vi "Symphony Setup V2.vi"(4 "areas :":i32[][](array[numeric])=[[1], [1], [1], [1024], [256], [1], [1]], 5 "Function":T1, 6 "Acq type":i32(ring)=1 items=["JYMCD_ACQ_FORMAT_IMAGE", "JYMCD_ACQ_FORMAT_SCAN"], 7 "Int_time(ms)":u16=10 caption="Integration time(ms)", 8 "error in (no error)":errorcluster, 9 "Gain":i32, 10 "Select ADC":i32(ring) items=["JY_ADC_16_BIT", "JY_ADC_14_BIT", "JY_ADC_18_BIT"], 11 "JYCCDLib.IJYCCDReqd":refnum<k7>) -> (0 "error out":errorcluster, 1 "DataSize":i32, 3 "JYCCDLib.IJYCCDReqdOut":refnum<k7>)   [LabVIEW 2019]
uses:
  AcqParState.ctl
panel:
  # "Area#"
  # "X Origin"
  # "Y Origin"
  # "X Size"
  # "Y Size"
  # "X Bin"
  # "Y Bin"
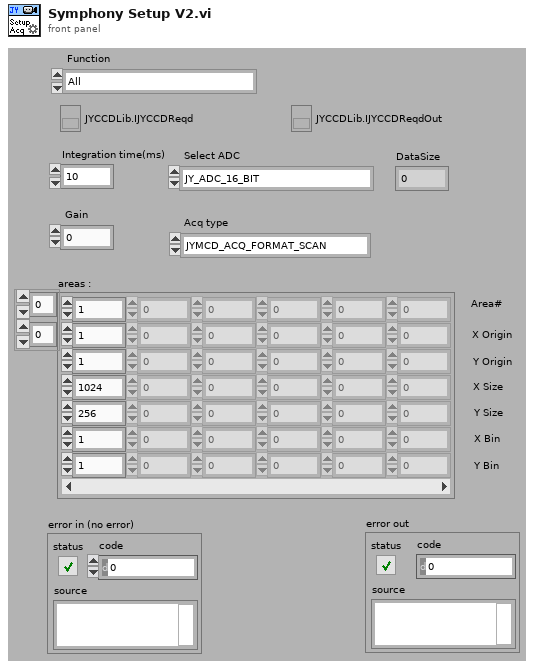
[diagram p1: front panel]
types:
  T1 = typedef "AcqParState.ctl" = enum16{"All", "ADC", "Gain", "AcqType", "IntegTime", "Areas", "Error"}
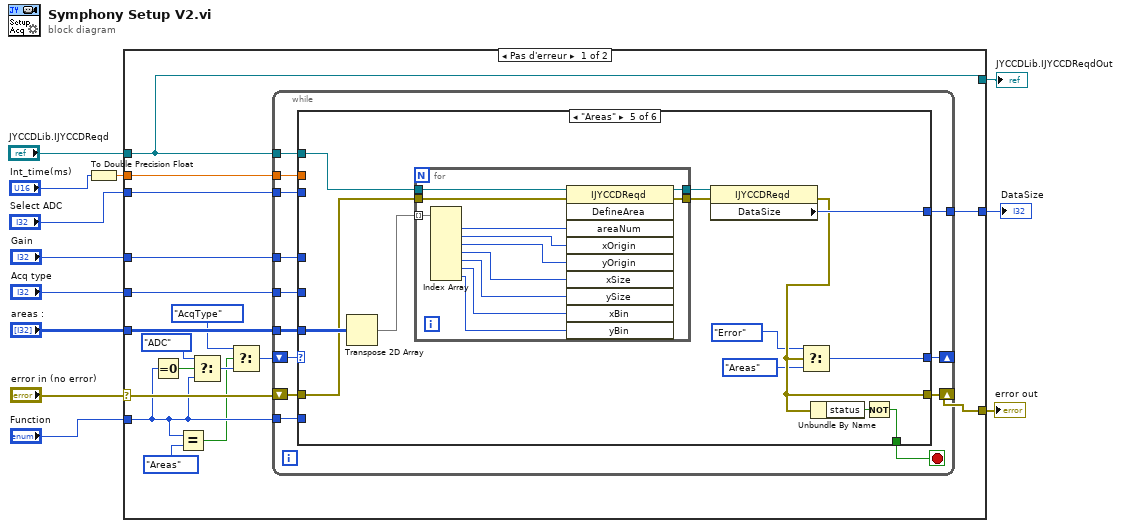
[diagram p0: block diagram]
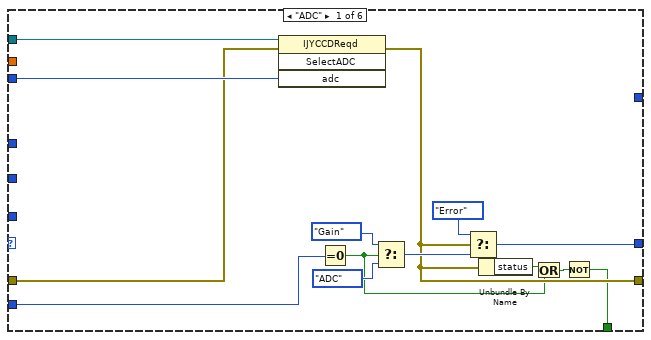
[diagram p2: hidden frame]
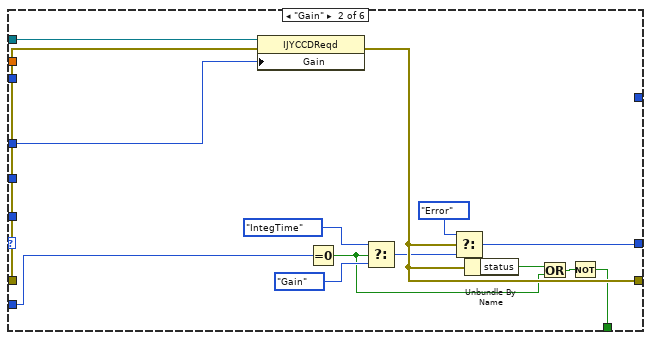
[diagram p3: hidden frame]
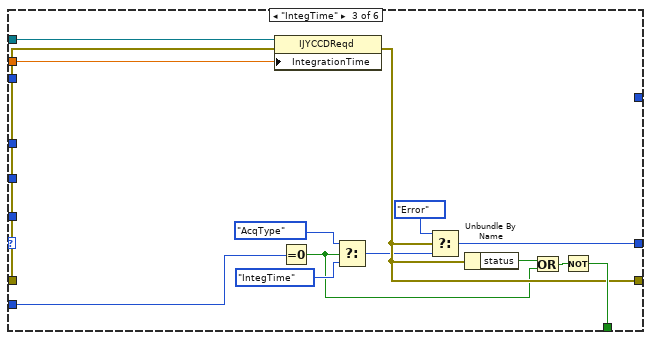
[diagram p4: hidden frame]
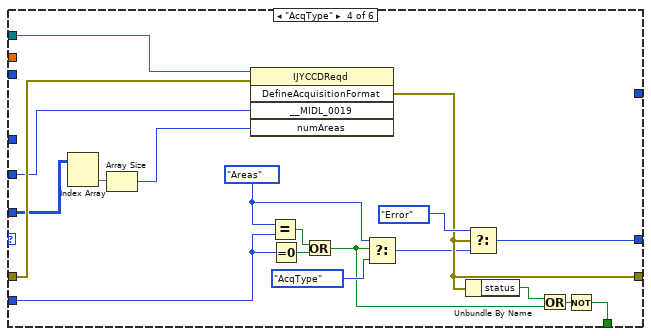
[diagram p5: hidden frame]
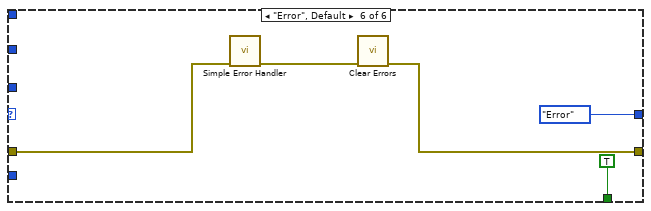
[diagram p6: hidden frame]
diagram:
  n1 = To Double Precision Float(number="Int_time(ms)") -> (double precision float=w8:dbl)
  n2 = case shown="Pas d'erreur" "error in (no error)" {
    selector: "error in (no error)" -> [w29 w135]
    tunnel: [w28 w135] -> w11
    tunnel: "JYCCDLib.IJYCCDReqd" -> [w25 w134]
    tunnel: w8 -> [w27 _]
    tunnel: "Select ADC" -> [w26 _]
    tunnel: [w25 w134] -> w6
    tunnel: "Gain" -> [w24 _]
    tunnel: "Acq type" -> [w23 _]
    tunnel: "areas :" -> [w22 _]
    tunnel: [w21 _] -> w2
    tunnel: "Function" -> [w17 _]
    frame No Error {
      n3 = Equal To 0?(x=w17) -> (x = 0?=w20:bool)
      n4 = Equal?(x=w17, y=AcqParState."Areas" ("Function")) -> (x = y?=w14:bool)
      n5 = Select(t=AcqParState."ADC" ("Function"), s=w20, f=w17) -> (s? t:f=w16:T1)
      n6 = Select(t=AcqParState."AcqType" ("Function"), s=w14, f=w16) -> (s? t:f=w15:T1)
      n7 = while {
        shift-right: [w38] -> w28
        shift-left: w29 -> [w41]
        tunnel: w25 -> [w42]
        shift-right: [w34] -> _
        shift-left: w15 -> [w30]
        tunnel: w27 -> [w40]
        tunnel: w26 -> [w39]
        tunnel: w24 -> [w37]
        tunnel: w23 -> [w36]
        tunnel: w22 -> [w35]
        tunnel: [w32] -> w21
        tunnel: w17 -> [w31]
        stop <- w33 stop-if-true
        n8 = case shown="\"Areas\"" w30 {
          tunnel: w42 -> [w53 w68 w83 w100 w105 _]
          tunnel: w41 -> [w54 w69 w84 w101 w104 w133]
          tunnel: w40 -> [_ _ w82 _ _ _]
          tunnel: w39 -> [w56 _ _ _ _ _]
          tunnel: [w47 w61 w76 w94 w109 w130] -> w38
          tunnel: w37 -> [_ w70 _ _ _ _]
          tunnel: w36 -> [_ _ _ w97 _ _]
          tunnel: w35 -> [_ _ _ w98 w108 _]
          tunnel: [w55 w58 w77 w103 w113 AcqParState."Error" ("Function")] -> w34
          tunnel: [w43 w57 w78 w102 w111 TRUE] -> w33
          tunnel: [_ _ _ _ w110 _] -> w32
          tunnel: w31 -> [w52 w66 w71 w90 _ _]
          frame "ADC" {
            n9 = invoke class="IJYCCDReqd" method="SelectADC"(reference=w53, error in=w54, "adc"=w56) -> (error out=w47:errorcluster)  [unwired: 1 in, 3 out]
            n10 = Equal To 0?(x=w52) -> (x = 0?=w45:bool)
            n11 = Select(t=AcqParState."Gain" ("Function"), s=w45, f=AcqParState."ADC" ("Function")) -> (s? t:f=w49:T1)
            n12 = Select(t=AcqParState."Error" ("Function"), s=w47, f=w49) -> (s? t:f=w55:T1)
            n13 = Unbundle By Name(w47) -> ("status"=w46:bool)
            n14 = Or(x=w46, y=w45) -> (x .or. y?=w44:bool)
            n15 = Not(x=w44) -> (.not. x?=w43:bool)
          }
          frame "Gain" {
            n16 = property class="IJYCCDReqd"(reference=w68, error in=w69, "Gain"=w70) -> (error out=w61:errorcluster)  [unwired: 1 out]
            n17 = Equal To 0?(x=w66) -> (x = 0?=w60:bool)
            n18 = Select(t=AcqParState."IntegTime" ("Function"), s=w60, f=AcqParState."Gain" ("Function")) -> (s? t:f=w59:T1)
            n19 = Select(t=AcqParState."Error" ("Function"), s=w61, f=w59) -> (s? t:f=w58:T1)
            n20 = Unbundle By Name(w61) -> ("status"=w63:bool)
            n21 = Or(x=w63, y=w60) -> (x .or. y?=w62:bool)
            n22 = Not(x=w62) -> (.not. x?=w57:bool)
          }
          frame "IntegTime" {
            n23 = property class="IJYCCDReqd"(reference=w83, error in=w84, "IntegrationTime"=w82) -> (error out=w76:errorcluster)  [unwired: 1 out]
            n24 = Equal To 0?(x=w71) -> (x = 0?=w73:bool)
            n25 = Select(t=AcqParState."AcqType" ("Function"), s=w73, f=AcqParState."IntegTime" ("Function")) -> (s? t:f=w72:T1)
            n26 = Select(t=AcqParState."Error" ("Function"), s=w76, f=w72) -> (s? t:f=w77:T1)
            n27 = Unbundle By Name(w76) -> ("status"=w80:bool)
            n28 = Or(x=w80, y=w73) -> (x .or. y?=w79:bool)
            n29 = Not(x=w79) -> (.not. x?=w78:bool)
          }
          frame "AcqType" {
            w91 = AcqParState."Areas" ("Function")
            n30 = Index Array(array=w98) -> (element=w99:i32[])  [unwired: 2 in]
            n31 = Array Size(array=w99) -> (size(s)=w96:i32)
            n32 = invoke class="IJYCCDReqd" method="DefineAcquisitionFormat"(reference=w100, error in=w101, "__MIDL_0019"=w97, "numAreas"=w96) -> (error out=w94:errorcluster)  [unwired: 1 in, 4 out]
            n33 = Equal?(x=w91, y=w90) -> (x = y?=w92:bool)
            n34 = Equal To 0?(x=w90) -> (x = 0?=w93:bool)
            n35 = Or(x=w92, y=w93) -> (x .or. y?=w87:bool)
            n36 = Select(t=w91, s=w87, f=AcqParState."AcqType" ("Function")) -> (s? t:f=w86:T1)
            n37 = Unbundle By Name(w94) -> ("status"=w85:bool)
            n38 = Select(t=AcqParState."Error" ("Function"), s=w94, f=w86) -> (s? t:f=w103:T1)
            n39 = Or(x=w85, y=w87) -> (x .or. y?=w88:bool)
            n40 = Not(x=w88) -> (.not. x?=w102:bool)
          }
          frame "Areas" {
            n41 = Transpose 2D Array(2D array=w108) -> (transposed array=w116:i32[][])
            n42 = for {
              tunnel: [w127] -> w114
              tunnel: [w126] -> w115
              tunnel: w116 -> [w125] mode=indexing
              tunnel: w104 -> [w118]
              tunnel: w105 -> [w117]
              n43 = Index Array(array=w125) -> (element #1=w128:i32, element #2=w124:i32, element #3=w123:i32, element #4=w122:i32, element #5=w121:i32, element #6=w120:i32, element #7=w119:i32)  [unwired: 7 in]
              n44 = invoke class="IJYCCDReqd" method="DefineArea"(reference=w117, error in=w118, "areaNum"=w128, "xOrigin"=w124, "yOrigin"=w123, "xSize"=w122, "ySize"=w121, "xBin"=w120, "yBin"=w119) -> (reference out=w127:refnum<k7>, error out=w126:errorcluster)  [unwired: 1 in, 8 out]
            }
            n45 = property class="IJYCCDReqd"(reference=w114, error in=w115) -> (error out=w109:errorcluster, "DataSize"=w110:i32)  [unwired: 1 out]
            n46 = Select(t=AcqParState."Error" ("Function"), s=w109, f=AcqParState."Areas" ("Function")) -> (s? t:f=w113:T1)
            n47 = Unbundle By Name(w109) -> ("status"=w112:bool)
            n48 = Not(x=w112) -> (.not. x?=w111:bool)
          }
          frame "Error", Default {
            n49 = call <vilib>:"Simple Error Handler.vi"("error in (no error)"=w133) -> ("error out"=w132:errorcluster)  [unwired: 4 in, 4 out]
            n50 = call <vilib>:"Clear Errors.vi"("error in (no error)"=w132) -> ("error out"=w130:errorcluster)  [unwired: 5 in, 1 out]
          }
        }
      }
    }
    frame Error {
    }
  }
  "DataSize" <- w2
  "JYCCDLib.IJYCCDReqdOut" <- w6
  "error out" <- w11
